vi "Setup Statically-Linked subWorkers.vi"(8 "error in":errorcluster, 11 "TCP Server in":refnum<class "DS TCP Server.lvclass">) -> (0 "error out":errorcluster, 3 "TCP Server out":refnum<class "DS TCP Server.lvclass">)   [LabVIEW 2017, in "DS TCP Server.lvlib" / "DS TCP Server.lvclass"]
doc: "<b>Note: Do not change the code in this VI!</b>\nThis VI performs a setup of all the statically-linked subWorkers that belong to the Worker that calls this VI. This VI is created automatically by the 'Create/Add Worker' tool and must be called <b>before</b> any statically linked subWorkers are called."
uses:
  DS TCP Server.lvclass
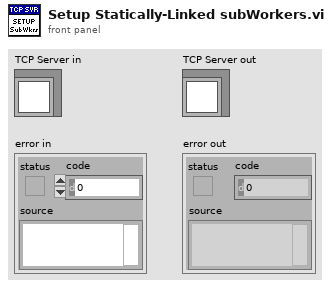
[diagram p1: front panel]
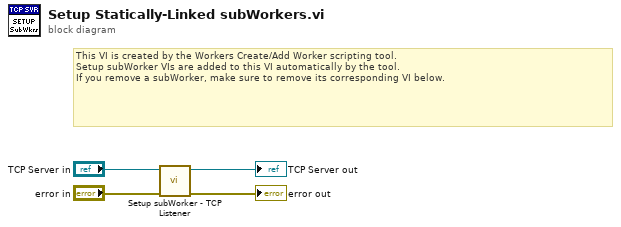
[diagram p0: block diagram]
diagram:
  # "This VI is created by the Workers Create/Add Worker scripting tool.\nSetup subWorker VIs are added to this VI automatically by the tool.\nIf you remove a subWorker, make sure to remove its corresponding VI below."
  n1 = call "Setup subWorker - TCP Listener.vi"("error in"="error in", "TCP Server in"="TCP Server in") -> ("error out"=→"error out":errorcluster, "TCP Server out"=→"TCP Server out":refnum<class "DS TCP Server.lvclass">)  [unwired: 8 in]
